vi "dfd_Calculate TapPerPhase.vi"(10 "factor":i32, 11 "#taps":i32) -> (3 "tapPerPhase":i32)   [LabVIEW 2017, in "NI_DigFilter_FXP.lvlib"]
uses:
  <vilib>/addons/Digital Filter Design/NI_DigFilter_FXP.lvlib
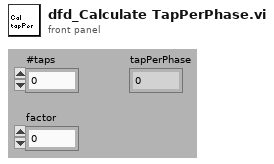
[diagram p1: front panel]
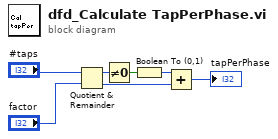
[diagram p0: block diagram]
diagram:
  n1 = Quotient & Remainder(x="#taps", y="factor") -> (x-y*floor(x/y)=w3:i32, floor(x/y)=w6:i32)
  n2 = Not Equal To 0?(x=w3) -> (x != 0?=w4:bool)
  n3 = Boolean To (0,1)(Boolean=w4) -> (0, 1=w5:i16)
  n4 = Add(x=w5, y=w6) -> (x+y=→"tapPerPhase":i32)
